vi "FTW-File-Extension.vi"(1 "Filepath":path) -> (0 "Extension":string)   [LabVIEW 2013]
panel:
  # "Inputs"
  # "Outputs"
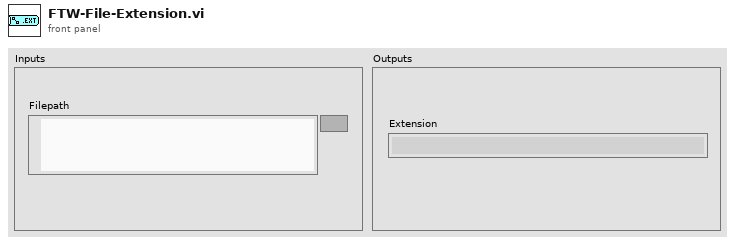
[diagram p1: front panel]
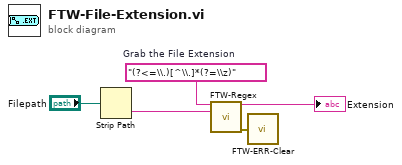
[diagram p0: block diagram]
diagram:
  w5 = "(?<=\\.)[^\\.]*(?=\\z)"  # Grab the File Extension
  n1 = Strip Path(path="Filepath") -> (name=w1:string)  [unwired: 1 out]
  n2 = call "FTW-Regex.vi"("Regular Expression"=w5, "Input String"=w1) -> ("Match"=→"Extension":string, "error out"=w4:errorcluster)  [unwired: 9 in, 3 out]
  n3 = call "FTW-ERR-Clear.vi"("error to snuff"=w4) -> ()  [unwired: 1 out]
